vi "Closest45rounding.vi"() -> ()   [LabVIEW 2018]
panel:
  out "NewAngle":dbl format="%#_13g"
  in  "Angle":dbl format="%#_13g"
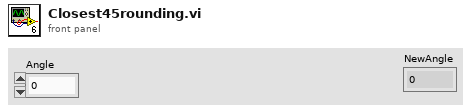
[diagram p1: front panel]
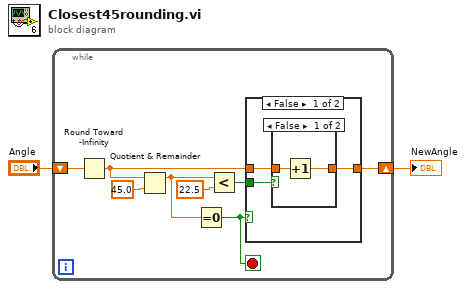
[diagram p0: block diagram]
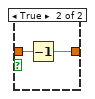
[diagram p2: hidden frame]
diagram:
  n1 = while {
    shift-right: [w9] -> w1
    shift-left: "Angle" -> [w8]
    stop <- w3 stop-if-true
    n2 = Round Toward -Infinity(1:w8) -> (0:w7:dbl)
    n3 = Quotient & Remainder(x=w7, y=45.0) -> (x-y*floor(x/y)=w5:dbl)  [unwired: 1 out]
    n4 = Equal To 0?(x=w5) -> (x = 0?=w3:bool)
    n5 = Less?(x=w5, y=22.5) -> (x < y?=w4:bool)
    n6 = case shown="False" w3 {
      tunnel: w7 -> [w13 w18]
      tunnel: [w12 w18] -> w9
      tunnel: w4 -> [w11 _]
      frame False {
        n7 = case shown="False" w11 {
          tunnel: w13 -> [w15 w17]
          tunnel: [w14 w16] -> w12
          frame False {
            n8 = Increment(x=w15) -> (x+1=w14:dbl)
          }
          frame True {
            n9 = Decrement(x=w17) -> (x-1=w16:dbl)
          }
        }
      }
      frame True {
      }
    }
  }
  "NewAngle" <- w1
